vi "Actor Core.vi"(8 "error in":errorcluster, 11 "DataLog in":refnum<class "Solutions.lvclass">) -> (0 "error out":errorcluster, 3 "Actor out":refnum<class "Actor.lvclass">)   [LabVIEW 2020, in "Test Forms.lvlib" / "Solutions.lvclass"]
doc: "The user interface for this panel.\n\n----\nPlease see the following web address for additional documentation and tutorial information:\nhttp://www.mooregoodideas.com/mgi-panel-manager/\n\nAuthor: Derek Trepanier\n\nCopyright (c) 2018, Moore Good Ideas, Inc.\n\nAll rights reserved.\n\nRedistribution and use in source and binary forms, with or without modification, are permitted provided that the following conditions are met:\n\n * Redistributions of source code must retain the above copyright notice, this list of conditions and the following disclaimer.\n * Redistributions in binary form must reproduce the above copyright notice, this list of conditions and the following disclaimer in the documentation and/or other materials provided with the distribution.\n * Neither the name of Moore Good Ideas, Inc. nor the names of its contributors may be used to endorse or promote products derived from this software without specific prior written permission.\n\nTHIS SOFTWARE IS PROVIDED BY THE COPYRIGHT HOLDERS AND CONTRIBUTORS \"AS IS\" AND ANY EXPRESS OR IMPLIED WARRANTIES, INCLUDING, BUT NOT LIMITED TO, THE IMPLIED WARRANTIES OF MERCHANTABILITY AND FITNESS FOR A PARTICULAR PURPOSE ARE DISCLAIMED. IN NO EVENT SHALL THE COPYRIGHT OWNER OR CONTRIBUTORS BE LIABLE FOR ANY DIRECT, INDIRECT, INCIDENTAL, SPECIAL, EXEMPLARY, OR CONSEQUENTIAL DAMAGES (INCLUDING, BUT NOT LIMITED TO, PROCUREMENT OF SUBSTITUTE GOODS OR SERVICES; LOSS OF USE, DATA, OR PROFITS; OR BUSINESS INTERRUPTION) HOWEVER CAUSED AND ON ANY THEORY OF LIABILITY, WHETHER IN CONTRACT, STRICT LIABILITY, OR TORT (INCLUDING NEGLIGENCE OR OTHERWISE) ARISING IN ANY WAY OUT OF THE USE OF THIS SOFTWARE, EVEN IF ADVISED OF THE POSSIBILITY OF SUCH DAMAGE."
uses:
  Solutions.lvclass
  C:/Users/User/Desktop/Raman Program/LV-Database-OOP/source/Forms AF/Forms Controller/Form Controller/Panel Form Controller.lvclass
  <vilib>/ActorFramework/Actor/Actor.lvclass
  Users/Users.lvclass
  source/Forms AF/Forms Controller/Form Controller/Panel Form Controller.lvclass/Panel Form Controller.ctl
  source/Forms AF/Forms Controller/Open Form Button/Open Form Button.lvclass
  C:/Users/User/Desktop/Raman Program/LV-Database-OOP/source/Database OOP/Button Libraries/Button Interface Class/Button Interface.lvclass
  source/Database OOP/Column Libraries/Basic Field Constructors/Text Field.vi
  source/Database OOP/Column Libraries/Basic Field Constructors/Numeric Field.vi
  source/Database OOP/Column Libraries/Basic Field Constructors/FK Ring Field.vi
  source/Database OOP/Column Libraries/Basic Field Constructors/Timestamp Field.vi
  source/Forms AF/Forms Controller/Form Window/Form Window.lvclass
  source/Database OOP/Table Libraries/Basic Form/Basic Form.lvclass
  source/Database OOP/Column Libraries/Composed Field Constructors.lvlib
  source/Forms AF/Forms Controller/Form Controller/Panel Form Controller.lvclass
panel:
  in  "pH":dbl
  in  "Date Made":timestamp
  in  "Description":string
  in  "Edit Users":bool
  in  "Short Name":string
  in  "User":u16(ring)
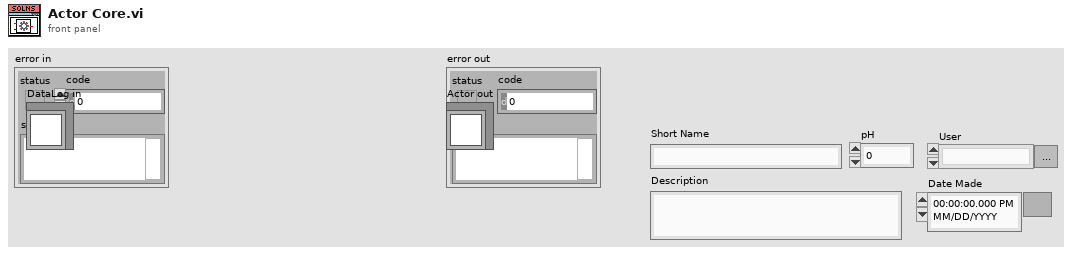
[diagram p1: front panel]
types:
  T1 = typedef "Panel Form Controller.lvlib/Builder Cluster.ctl" = cluster{"VI Ctrl Array":refnum<vi>[], "Form":refnum<class "Basic Form.lvclass">, "Open Form Button":refnum<class "Open Form Button.lvclass">}
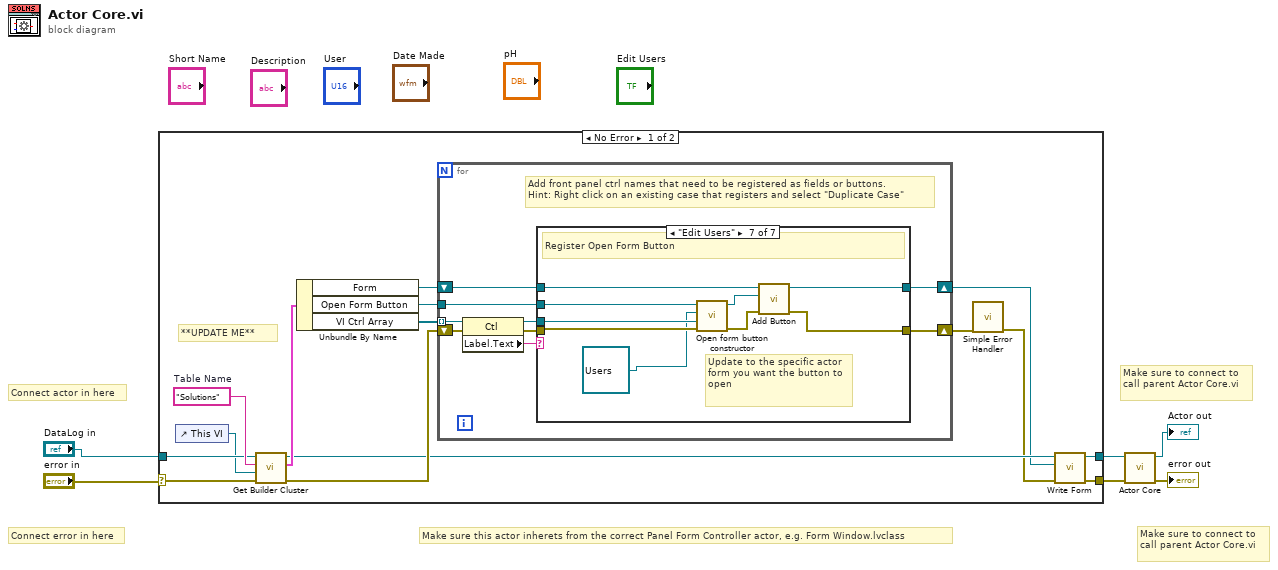
[diagram p0: block diagram]
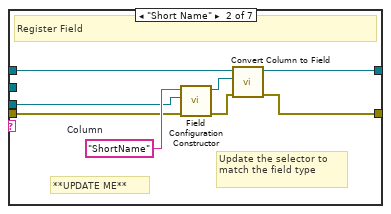
[diagram p3: hidden frame]
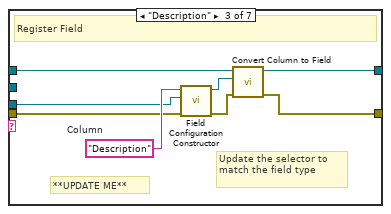
[diagram p4: hidden frame]
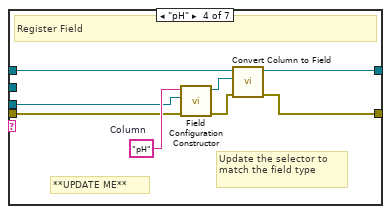
[diagram p5: hidden frame]
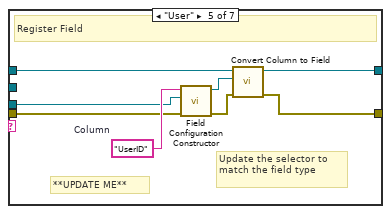
[diagram p6: hidden frame]
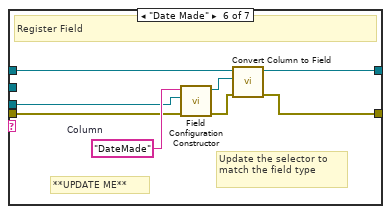
[diagram p7: hidden frame]
diagram:
  # "Make sure to connect to\ncall parent Actor Core.vi"
  # "Make sure to connect to\ncall parent Actor Core.vi"
  # "Make sure this actor inherets from the correct Panel Form Controller actor, e.g. Form Window.lvclass"
  # "Connect error in here"
  # "Connect actor in here"
  n1 = case shown="No Error" "error in" {
    selector: "error in" -> [w18 w83]
    tunnel: "DataLog in" -> [w8 w82]
    tunnel: [w12 w83] -> w3
    tunnel: [w13 w82] -> w4
    frame No Error {
      w11 = "Solutions"  # Table Name
      # "**UPDATE ME**"
      n2 = control-ref of="This VI"() -> (w7:refnum<vi>)
      n3 = call "Get Builder Cluster.vi"("error in (no error)"=w18, "VI Refnum"=w7, "Table Name"=w11, "Panel Form Controller in"=w8) -> ("error out"=w20:errorcluster, "Builder Cluster"=w19:T1, "Panel Form Controller out"=w15:refnum<class "Solutions.lvclass">)  [unwired: 5 in]
      n4 = Unbundle By Name(w19) -> ("Form"=w21:refnum<class "Basic Form.lvclass">, "Open Form Button"=w16:refnum<class "Open Form Button.lvclass">, "VI Ctrl Array"=w17:refnum<vi>[])
      n5 = for {
        tunnel: w17 -> [w30] mode=indexing
        shift-right: [w24] -> w14
        shift-left: w21 -> [w25]
        shift-right: [w22] -> w10
        shift-left: w20 -> [w28]
        tunnel: w16 -> [w23]
        # "Add front panel ctrl names that need to be registered as fields or buttons.\nHint: Right click on an existing case that registers and select \"Duplicate Case\""
        n6 = property class="Ctl"(reference=w30, error in=w28) -> (reference out=w29:refnum<vi>, error out=w27:errorcluster, "Label.Text"=w26:string)
        n7 = case shown="\"Edit Users\"" w26 {
          tunnel: w29 -> [_ w35 w43 w51 w59 w67 w75]
          tunnel: w25 -> [w32 w40 w48 w56 w64 w72 w81]
          tunnel: [w32 w38 w46 w54 w62 w70 w80] -> w24
          tunnel: [w31 w39 w47 w55 w63 w71 w79] -> w22
          tunnel: w27 -> [w31 w34 w42 w50 w58 w66 w74]
          tunnel: w23 -> [_ _ _ _ _ _ w76]
          frame "", Default {
            # "Not Registered"
          }
          frame "Short Name" {
            w36 = "ShortName"  # Column
            # "Update the selector to match the field type"
            # "**UPDATE ME**"
            # "Register Field"
            n8 = call-poly "Field Configuration Constructor.vi"("error in"=w34, "Ctl Refnum"=w35, "Column Name"=w36) -> ("error out"=w37:errorcluster, "Field Configuration"=w33:refnum<class "Field Configuration.lvclass">)  [unwired: 7 in]
            n9 = call "Convert Column to Field.vi"("error in (no error)"=w37, "Field Configuration"=w33, "Basic Form in"=w40) -> ("error out"=w39:errorcluster, "Basic Form out"=w38:refnum<class "Basic Form.lvclass">)  [unwired: 7 in]
          }
          frame "Description" {
            w44 = "Description"  # Column
            # "Update the selector to match the field type"
            # "**UPDATE ME**"
            # "Register Field"
            n10 = call-poly "Field Configuration Constructor.vi"("error in"=w42, "Ctl Refnum"=w43, "Column Name"=w44) -> ("error out"=w45:errorcluster, "Field Configuration"=w41:refnum<class "Field Configuration.lvclass">)  [unwired: 7 in]
            n11 = call "Convert Column to Field.vi"("error in (no error)"=w45, "Field Configuration"=w41, "Basic Form in"=w48) -> ("error out"=w47:errorcluster, "Basic Form out"=w46:refnum<class "Basic Form.lvclass">)  [unwired: 7 in]
          }
          frame "pH" {
            w52 = "pH"  # Column
            # "Update the selector to match the field type"
            # "**UPDATE ME**"
            # "Register Field"
            n12 = call-poly "Field Configuration Constructor.vi"("error in"=w50, "Ctl Refnum"=w51, "Column Name"=w52) -> ("error out"=w53:errorcluster, "Field Configuration"=w49:refnum<class "Field Configuration.lvclass">)  [unwired: 7 in]
            n13 = call "Convert Column to Field.vi"("error in (no error)"=w53, "Field Configuration"=w49, "Basic Form in"=w56) -> ("error out"=w55:errorcluster, "Basic Form out"=w54:refnum<class "Basic Form.lvclass">)  [unwired: 7 in]
          }
          frame "User" {
            w60 = "UserID"  # Column
            # "Update the selector to match the field type"
            # "**UPDATE ME**"
            # "Register Field"
            n14 = call-poly "Field Configuration Constructor.vi"("error in"=w58, "Ctl Refnum"=w59, "Column Name"=w60) -> ("error out"=w61:errorcluster, "Field Configuration"=w57:refnum<class "Field Configuration.lvclass">)  [unwired: 7 in]
            n15 = call "Convert Column to Field.vi"("error in (no error)"=w61, "Field Configuration"=w57, "Basic Form in"=w64) -> ("error out"=w63:errorcluster, "Basic Form out"=w62:refnum<class "Basic Form.lvclass">)  [unwired: 7 in]
          }
          frame "Date Made" {
            w68 = "DateMade"  # Column
            # "Update the selector to match the field type"
            # "**UPDATE ME**"
            # "Register Field"
            n16 = call-poly "Field Configuration Constructor.vi"("error in"=w66, "Ctl Refnum"=w67, "Column Name"=w68) -> ("error out"=w69:errorcluster, "Field Configuration"=w65:refnum<class "Field Configuration.lvclass">)  [unwired: 7 in]
            n17 = call "Convert Column to Field.vi"("error in (no error)"=w69, "Field Configuration"=w65, "Basic Form in"=w72) -> ("error out"=w71:errorcluster, "Basic Form out"=w70:refnum<class "Basic Form.lvclass">)  [unwired: 7 in]
          }
          frame "Edit Users" {
            # "Update to the specific actor form you want the button to open"
            # "Register Open Form Button"
            n18 = call "Open form button constructor.vi"("error in (no error)"=w74, "Ctl Refnum"=w75, "Panel Form"=refnum<class "Users.lvclass"> refnum ("Test Forms.lvlib:Users.lvclass"), "Open Form Button in"=w76) -> ("error out"=w77:errorcluster, "Open Form Button out"=w78:refnum<class "Open Form Button.lvclass">)  [unwired: 6 in]
            n19 = call "Add Button.vi"("error in (no error)"=w77, "Button"=w78, "Basic Form in"=w81) -> ("error out"=w79:errorcluster, "Basic Form out"=w80:refnum<class "Basic Form.lvclass">)  [unwired: 7 in]
          }
        }
      }
      n20 = call <vilib>:"Simple Error Handler.vi"("error in (no error)"=w10) -> ("error out"=w9:errorcluster)  [unwired: 4 in, 4 out]
      n21 = call "Write Form.vi"("error in (no error)"=w9, "Form.lvlib:Basic Form.lvclass"=w14, "Panel Form Controller in"=w15) -> ("error out"=w12:errorcluster, "Panel Form Controller out"=w13:refnum<class "Solutions.lvclass">)  [unwired: 7 in]
    }
    frame Error {
    }
  }
  n22 = call-parent "Actor Core.vi"("error in"=w3, "Form Window in"=w4) -> ("error out"=→"error out":errorcluster, "Actor out"=→"Actor out":refnum<class "Actor.lvclass">)  [unwired: 8 in]
